vi "Tutorial 11.vi"() -> ()   [LabVIEW 2014]
panel:
  out "Square Root of X":dbl
  in  "Number X":dbl
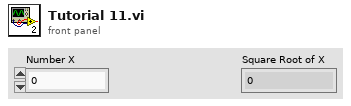
[diagram p1: front panel]
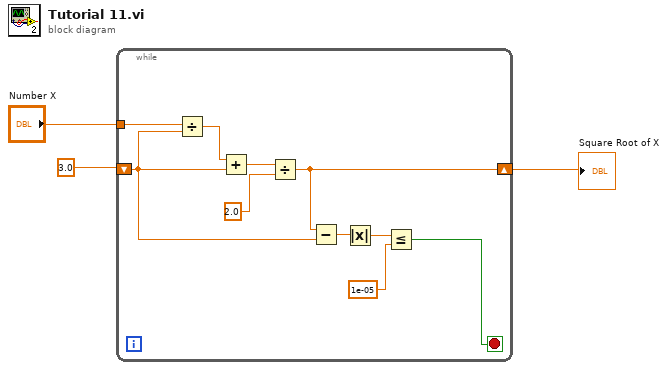
[diagram p0: block diagram]
diagram:
  n1 = while {
    tunnel: "Number X" -> [w13]
    shift-right: [w9] -> w1
    shift-left: 3.0 -> [w8]
    stop <- w4 stop-if-true
    n2 = Divide(x=w13, y=w8) -> (x/y=w12:dbl)
    n3 = Add(x=w12, y=w8) -> (x+y=w11:dbl)
    n4 = Divide(x=w11, y=2.0) -> (x/y=w9:dbl)
    n5 = Subtract(x=w9, y=w8) -> (x-y=w7:dbl)
    n6 = Absolute Value(x=w7) -> (abs(x)=w6:dbl)
    n7 = Less Or Equal?(x=w6, y=1e-05) -> (x <= y?=w4:bool)
  }
  "Square Root of X" <- w1
